vi "Get Timing Information.vi"(8 "error in (no error)":errorcluster, 11 "DSFTiming in":refnum<class "DSFTiming.lvclass">) -> (0 "error out":errorcluster, 2 "timing info":T1, 3 "DSFTiming out":refnum<class "DSFTiming.lvclass">)   [LabVIEW 2017, in "DSFTiming.lvclass"]
uses:
  DSFTiming.lvclass
  Controls/dsf timing.ctl
  DSFTiming.lvclass/DSFTiming.ctl
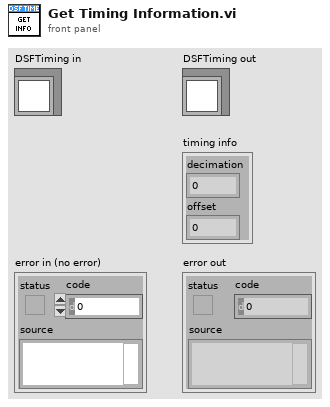
[diagram p1: front panel]
types:
  T1 = typedef "dsf timing.ctl" = cluster{"decimation":i32, "offset":i32}
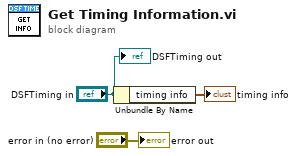
[diagram p0: block diagram]
diagram:
  n1 = Unbundle By Name("DSFTiming in") -> ("timing info"=→"timing info":T1)
  "error out" <- "error in (no error)"
  "DSFTiming out" <- "DSFTiming in"
